vi "Send Pulse Instructions.vi"(8 "error in":errorcluster, 11 "3300 in":refnum<class "3300.lvclass">) -> (0 "error out":errorcluster, 3 "3300 out":refnum<class "3300.lvclass">)   [LabVIEW 2019, in "3300.lvlib" / "3300.lvclass"]
uses:
  Library/3300.lvclass
  C:/Users/Public/Documents/Development/builds/Instruments/Electronic Load.lvlibp/Library/Electronic Load.lvclass
  builds/Instruments/Electronic Load.lvlibp/Accessors/Trigger/Read Pulse Enable.vi
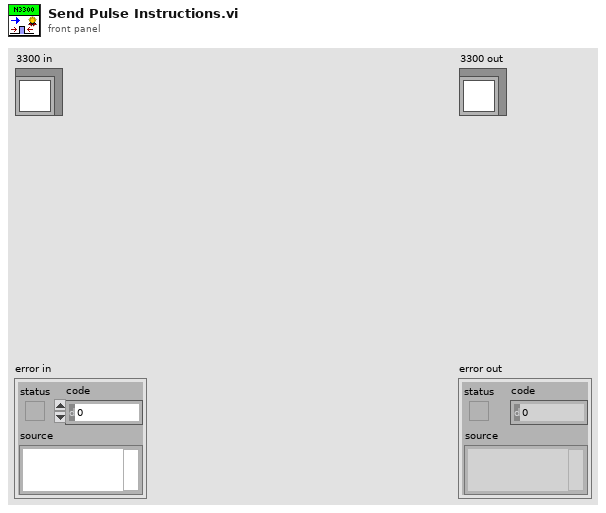
[diagram p1: front panel]
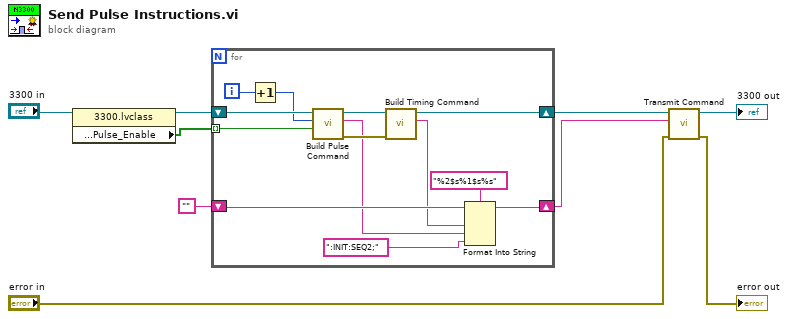
[diagram p0: block diagram]
diagram:
  n1 = property class="3300.lvclass"(reference="3300 in") -> (reference out=w8:refnum<class "3300.lvclass">, "Accessors:Settings:Pulse:Pulse_Enable"=w6:bool[])  [unwired: 1 in, 1 out]
  n2 = for {
    shift-right: [w18] -> w5
    shift-left: w8 -> [w19]
    shift-right: [w21] -> w1
    shift-left: "" -> [w22]
    tunnel: w6 -> [w11] mode=indexing
    i -> [w13]
    n3 = Increment(x=w13) -> (x+1=w12:i32)
    n4 = call "Build Pulse Command.vi"("Pulse Enable"=w11, "Channel"=w12, "3300 in"=w19) -> ("error out"=w17:errorcluster, "Pulse Instruction"=w16:string, "3300 out"=w20:refnum<class "3300.lvclass">)  [unwired: 6 in]
    n5 = call "Build Timing Command.vi"("error in"=w17, "3300 in"=w20) -> ("resulting string"=w15:string, "3300 out"=w18:refnum<class "3300.lvclass">)  [unwired: 7 in, 1 out]
    n6 = Format Into String(format string="%2$s%1$s%s", initial string=w22, w15, w16, ":INIT:SEQ2;" ("format string")) -> (resulting string=w21:string)  [unwired: 1 in, 1 out]
  }
  n7 = call "Transmit Command.vi"("error in"="error in", "Command"=w1, "3300 in"=w5) -> ("error out"=→"error out":errorcluster, "3300 out"=→"3300 out":refnum<class "3300.lvclass">)  [unwired: 7 in]
